vi "InitConfig.vi"   [LabVIEW 2011]
uses:
  <vilib>/Utility/config.llb/Write Key (Double).vi
  <vilib>/Utility/config.llb/Write Key (I32).vi
  <vilib>/Utility/config.llb/Write Key (String).vi
  <vilib>/Utility/config.llb/NI_LVConfig.lvlib
types:
  T1 = typedef "NI_LVConfig.lvlib/Config Data RefNum.ctl" = refnum<k1>
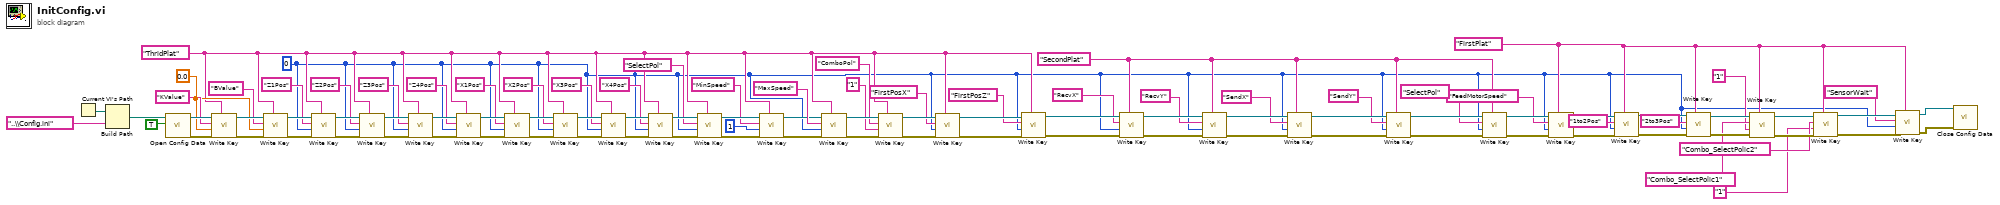
[diagram p0: block diagram]
diagram:
  w5 = "FirstPlat" ("section")
  w26 = "SecondPlat" ("section")
  w3 = 0
  w44 = "ThridPlat" ("section")
  w62 = 0.0
  n1 = Current VI's Path() -> (path=w96:path)
  n2 = Build Path(base path=w96, name or relative path="..\\Config.ini" ("名称或相对路径")) -> (appended path=w94:path)
  n3 = call <vilib>:"Open Config Data.vi"("create file if necessary (T)"=TRUE, "configuration file path"=w94) -> ("error out"=w90:errorcluster, "refnum"=w92:T1)  [unwired: 7 in, 1 out]
  n4 = call-poly <vilib>:"Write Key.vi"("section"=w44, "error in (no error)"=w90, "value"=w62, "key"="KValue", "refnum"=w92) -> ("error out"=w88:errorcluster, "refnum out"=w89:T1)  [unwired: 4 in, 1 out]
  n5 = call-poly <vilib>:"Write Key.vi"("section"=w44, "error in (no error)"=w88, "value"=w62, "key"="BValue", "refnum"=w89) -> ("error out"=w86:errorcluster, "refnum out"=w85:T1)  [unwired: 4 in, 1 out]
  n6 = call-poly <vilib>:"Write Key.vi"("section"=w44, "error in (no error)"=w86, "value"=w3, "key"="Z1Pos", "refnum"=w85) -> ("error out"=w83:errorcluster, "refnum out"=w82:T1)  [unwired: 4 in, 1 out]
  n7 = call-poly <vilib>:"Write Key.vi"("section"=w44, "error in (no error)"=w83, "value"=w3, "key"="Z2Pos", "refnum"=w82) -> ("error out"=w80:errorcluster, "refnum out"=w81:T1)  [unwired: 4 in, 1 out]
  n8 = call-poly <vilib>:"Write Key.vi"("section"=w44, "error in (no error)"=w80, "value"=w3, "key"="Z3Pos", "refnum"=w81) -> ("error out"=w78:errorcluster, "refnum out"=w79:T1)  [unwired: 4 in, 1 out]
  n9 = call-poly <vilib>:"Write Key.vi"("section"=w44, "error in (no error)"=w78, "value"=w3, "key"="Z4Pos", "refnum"=w79) -> ("error out"=w76:errorcluster, "refnum out"=w77:T1)  [unwired: 4 in, 1 out]
  n10 = call-poly <vilib>:"Write Key.vi"("section"=w44, "error in (no error)"=w76, "value"=w3, "key"="X1Pos", "refnum"=w77) -> ("error out"=w74:errorcluster, "refnum out"=w75:T1)  [unwired: 4 in, 1 out]
  n11 = call-poly <vilib>:"Write Key.vi"("section"=w44, "error in (no error)"=w74, "value"=w3, "key"="X2Pos", "refnum"=w75) -> ("error out"=w72:errorcluster, "refnum out"=w73:T1)  [unwired: 4 in, 1 out]
  n12 = call-poly <vilib>:"Write Key.vi"("section"=w44, "error in (no error)"=w72, "value"=w3, "key"="X3Pos", "refnum"=w73) -> ("error out"=w70:errorcluster, "refnum out"=w71:T1)  [unwired: 4 in, 1 out]
  n13 = call-poly <vilib>:"Write Key.vi"("section"=w44, "error in (no error)"=w70, "value"=w3, "key"="X4Pos", "refnum"=w71) -> ("error out"=w60:errorcluster, "refnum out"=w61:T1)  [unwired: 4 in, 1 out]
  n14 = call-poly <vilib>:"Write Key.vi"("section"=w44, "error in (no error)"=w60, "value"=w3, "key"="SelectPol", "refnum"=w61) -> ("error out"=w58:errorcluster, "refnum out"=w59:T1)  [unwired: 4 in, 1 out]
  n15 = call-poly <vilib>:"Write Key.vi"("section"=w44, "error in (no error)"=w58, "value"=1, "key"="MinSpeed", "refnum"=w59) -> ("error out"=w53:errorcluster, "refnum out"=w54:T1)  [unwired: 4 in, 1 out]
  n16 = call-poly <vilib>:"Write Key.vi"("section"=w44, "error in (no error)"=w53, "value"=w3, "key"="MaxSpeed", "refnum"=w54) -> ("error out"=w51:errorcluster, "refnum out"=w52:T1)  [unwired: 4 in, 1 out]
  n17 = call-poly <vilib>:"Write Key.vi"("section"=w44, "error in (no error)"=w51, "value"="1", "key"="ComboPol", "refnum"=w52) -> ("error out"=w46:errorcluster, "refnum out"=w47:T1)  [unwired: 4 in, 1 out]
  n18 = call-poly <vilib>:"Write Key.vi"("section"=w44, "error in (no error)"=w46, "value"=w3, "key"="FirstPosX", "refnum"=w47) -> ("error out"=w42:errorcluster, "refnum out"=w43:T1)  [unwired: 4 in, 1 out]
  n19 = call-poly <vilib>:"Write Key.vi"("section"=w44, "error in (no error)"=w42, "value"=w3, "key"="FirstPosZ", "refnum"=w43) -> ("error out"=w38:errorcluster, "refnum out"=w40:T1)  [unwired: 4 in, 1 out]
  n20 = call-poly <vilib>:"Write Key.vi"("section"=w26, "error in (no error)"=w38, "value"=w3, "key"="RecvX", "refnum"=w40) -> ("error out"=w37:errorcluster, "refnum out"=w36:T1)  [unwired: 4 in, 1 out]
  n21 = call-poly <vilib>:"Write Key.vi"("section"=w26, "error in (no error)"=w37, "value"=w3, "key"="RecvY", "refnum"=w36) -> ("error out"=w33:errorcluster, "refnum out"=w34:T1)  [unwired: 4 in, 1 out]
  n22 = call-poly <vilib>:"Write Key.vi"("section"=w26, "error in (no error)"=w33, "value"=w3, "key"="SendX", "refnum"=w34) -> ("error out"=w31:errorcluster, "refnum out"=w32:T1)  [unwired: 4 in, 1 out]
  n23 = call-poly <vilib>:"Write Key.vi"("section"=w26, "error in (no error)"=w31, "value"=w3, "key"="SendY", "refnum"=w32) -> ("error out"=w28:errorcluster, "refnum out"=w27:T1)  [unwired: 4 in, 1 out]
  n24 = call-poly <vilib>:"Write Key.vi"("section"=w26, "error in (no error)"=w28, "value"=w3, "key"="SelectPol", "refnum"=w27) -> ("error out"=w23:errorcluster, "refnum out"=w24:T1)  [unwired: 4 in, 1 out]
  n25 = call-poly <vilib>:"Write Key.vi"("section"=w5, "error in (no error)"=w23, "value"=w3, "key"="FeedMotorSpeed", "refnum"=w24) -> ("error out"=w20:errorcluster, "refnum out"=w21:T1)  [unwired: 4 in, 1 out]
  n26 = call-poly <vilib>:"Write Key.vi"("section"=w5, "error in (no error)"=w20, "value"=w3, "key"="1to2Pos", "refnum"=w21) -> ("error out"=w17:errorcluster, "refnum out"=w18:T1)  [unwired: 4 in, 1 out]
  n27 = call-poly <vilib>:"Write Key.vi"("section"=w5, "error in (no error)"=w17, "value"=w3, "key"="2to3Pos", "refnum"=w18) -> ("error out"=w14:errorcluster, "refnum out"=w15:T1)  [unwired: 4 in, 1 out]
  n28 = call-poly <vilib>:"Write Key.vi"("section"=w5, "error in (no error)"=w14, "value"="1" ("key"), "key"="Combo_SelectPolic1", "refnum"=w15) -> ("error out"=w10:errorcluster, "refnum out"=w11:T1)  [unwired: 4 in, 1 out]
  n29 = call-poly <vilib>:"Write Key.vi"("section"=w5, "error in (no error)"=w10, "value"="1" ("key"), "key"="Combo_SelectPolic2", "refnum"=w11) -> ("error out"=w6:errorcluster, "refnum out"=w7:T1)  [unwired: 4 in, 1 out]
  n30 = call-poly <vilib>:"Write Key.vi"("section"=w5, "error in (no error)"=w6, "value"=w3, "key"="SensorWait", "refnum"=w7) -> ("error out"=w1:errorcluster, "refnum out"=w2:T1)  [unwired: 4 in, 1 out]
  n31 = call <vilib>:"Close Config Data.vi"("error in (no error)"=w1, "refnum"=w2) -> ()  [unwired: 1 in, 9 out]
